vi "ParamsFasor.vi"(2 "paramsIn":variant) -> (16 "paramsOut":variant)   [LabVIEW 2017]
uses:
  Typedefs/Tipo_ParamsFasor.ctl
panel:
  in  "Amplitude Pulso":dbl
  in  "Largura Pulsos (ms)":dbl
  in  "Freq. Pulsos (Hz)":dbl
  in  "Init":bool
  in  "Amplitude Repouso":dbl
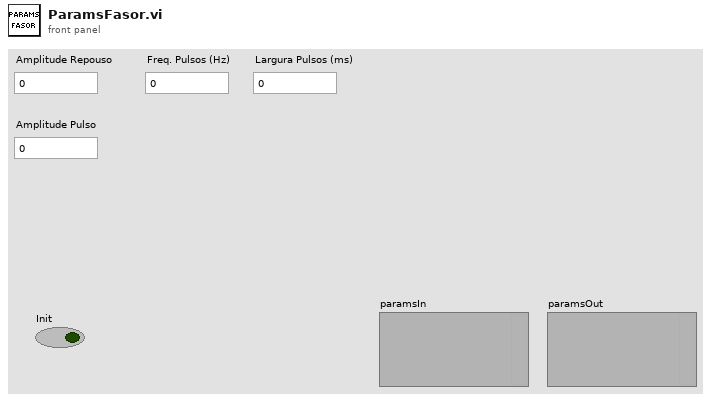
[diagram p1: front panel]
types:
  T1 = typedef "Tipo_ParamsFasor.ctl" = cluster{"Amplitude Repouso":dbl, "Amplitude Pulso":dbl, "Freq. Pulsos":dbl, "Largura Pulsos":dbl}
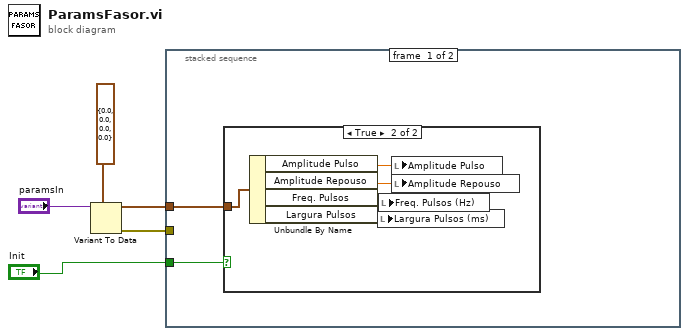
[diagram p0: block diagram]
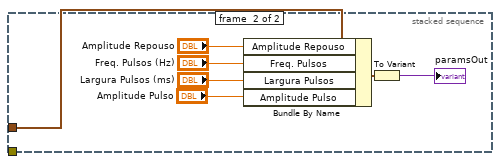
[diagram p3: hidden frame]
diagram:
  n1 = Variant To Data(type=T1 {"Amplitude Repouso"=0.0, "Amplitude Pulso"=0.0, "Freq. Pulsos"=0.0, "Largura Pulsos"=0.0} ("ParamsIn"), Variant="paramsIn") -> (data=w3:T1, error out=w1:errorcluster)  [unwired: 1 in]
  n2 = stacked-sequence {
    tunnel: w3 -> [w7 w19]
    tunnel: "Init" -> [w6 _]
    tunnel: w1 -> [_ _]
    frame #0 {
      n3 = case shown="True" w6 {
        tunnel: w7 -> [_ w12]
        frame False {
        }
        frame True {
          n4 = Unbundle By Name(w12) -> ("Amplitude Pulso"=w8:dbl, "Amplitude Repouso"=w11:dbl, "Freq. Pulsos"=w10:dbl, "Largura Pulsos"=w9:dbl)
          n5 = local write "Largura Pulsos (ms)"(w9) -> ()
          n6 = local write "Freq. Pulsos (Hz)"(w10) -> ()
          n7 = local write "Amplitude Pulso"(w8) -> ()
          n8 = local write "Amplitude Repouso"(w11) -> ()
        }
      }
    }
    frame #1 {
      n9 = Bundle By Name(cluster=w19, "Amplitude Repouso"="Amplitude Repouso", "Freq. Pulsos"="Freq. Pulsos (Hz)", "Largura Pulsos"="Largura Pulsos (ms)", "Amplitude Pulso"="Amplitude Pulso") -> (w17:T1)
      n10 = To Variant(anything=w17) -> (Variant=→"paramsOut":variant)
    }
  }
